vi "Close.vi"(8 "error in (no error)":errorcluster, 11 "PI Relays in":refnum<class "PI Relays.lvclass">) -> (0 "error out":errorcluster, 3 "PI Relays out":refnum<class "PI Relays.lvclass">)   [LabVIEW 2020, in "PI Relays.lvlib" / "PI Relays.lvclass"]
uses:
  PI Relays.lvclass
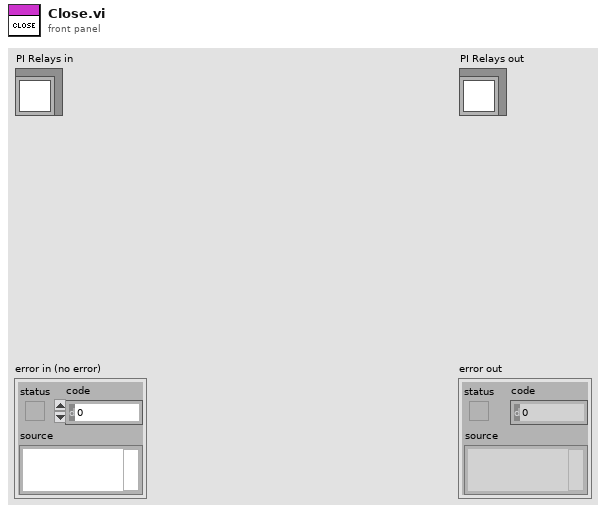
[diagram p1: front panel]
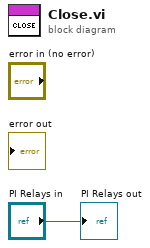
[diagram p0: block diagram]
diagram:
  "PI Relays out" <- "PI Relays in"
